vi "Pockels sequence gen-lines.vi"(8 "error in (no error)":errorcluster) -> (0 "error out":errorcluster, 1 "Lines in chunk for the trigger period target (ms)":i32, 3 "Ref Scan Cycles":i32)   [LabVIEW 2017]
uses:
  Typedefs/Pockels modulation setup cluster.ctl
  Typedefs/Frame Size.ctl
  Globals/gl_Pockels control globals.vi
panel:
  in  "Use simulation input cluster below":bool
  in  "Input values cluster":T1={"Frame Size"=512, "Fill time (us)"=24.5, "Dwell time (us)"=0.1} {"Dwell time (us)" format="%#_13g"; "Fill time (us)" format="%#_13g"; "Frame Size" items=["100X100"=100, "128X128"=128, "200X200"=200, "256X256"=256, "512X512"=512, "1024x1024"=1024, "2048x2048"=2048]}
  out "time between reference triggers (ms)":dbl[](array[numeric])
  out "Time for main img line (ms)":dbl
  out "time length of each chunk (ms)":dbl[](array[numeric])
  out "Number of lines in each chunk":i32[](array[numeric]) format="%.0f lines each"
  out "Chunks":i32[](array[numeric]) format="%.0f chunks of"
  out "Adjusted time between ref \ntriggers sent to the FPGA (ms)":dbl format="%#_10g"
  out "Actual resulting time between ref triggers (ms)":dbl format="%#_10g"
  # "INPUTS"
  # "INFORMATION"
  # "Possible combinations resulting in a number of chunks with equal number of lines"
  # "+ Time for ref image"
  # "OUTPUTS"
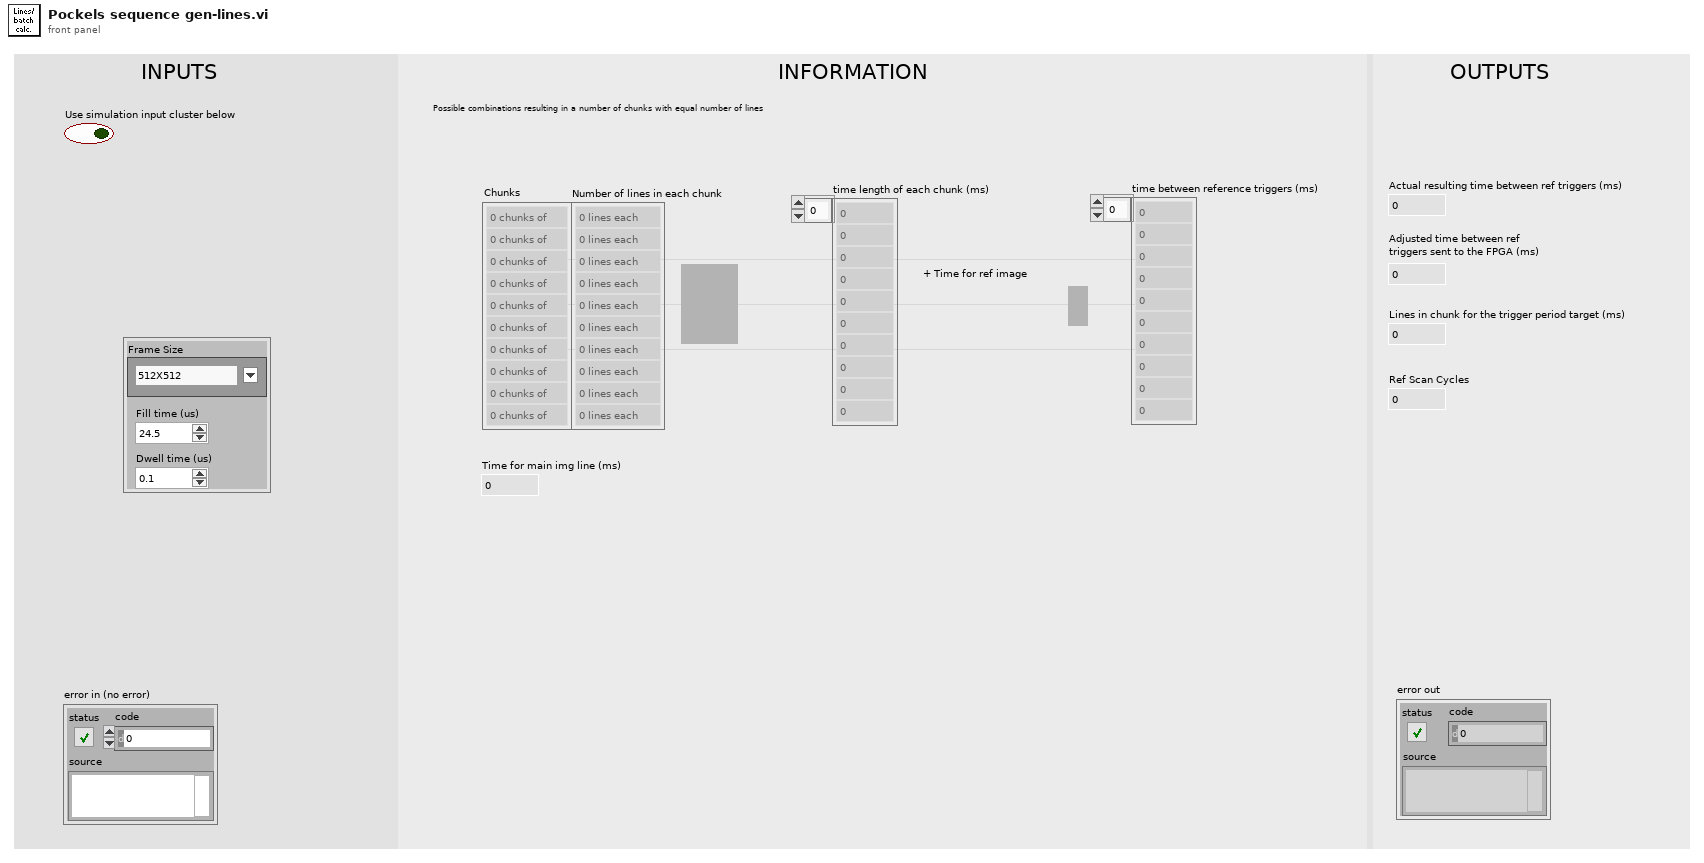
[diagram p1: front panel]
types:
  T1 = typedef "Pockels modulation setup cluster.ctl" = cluster{"Frame Size":T2, "Fill time (us)":dbl, "Dwell time (us)":dbl}
  T2 = typedef "Frame Size.ctl" = u16
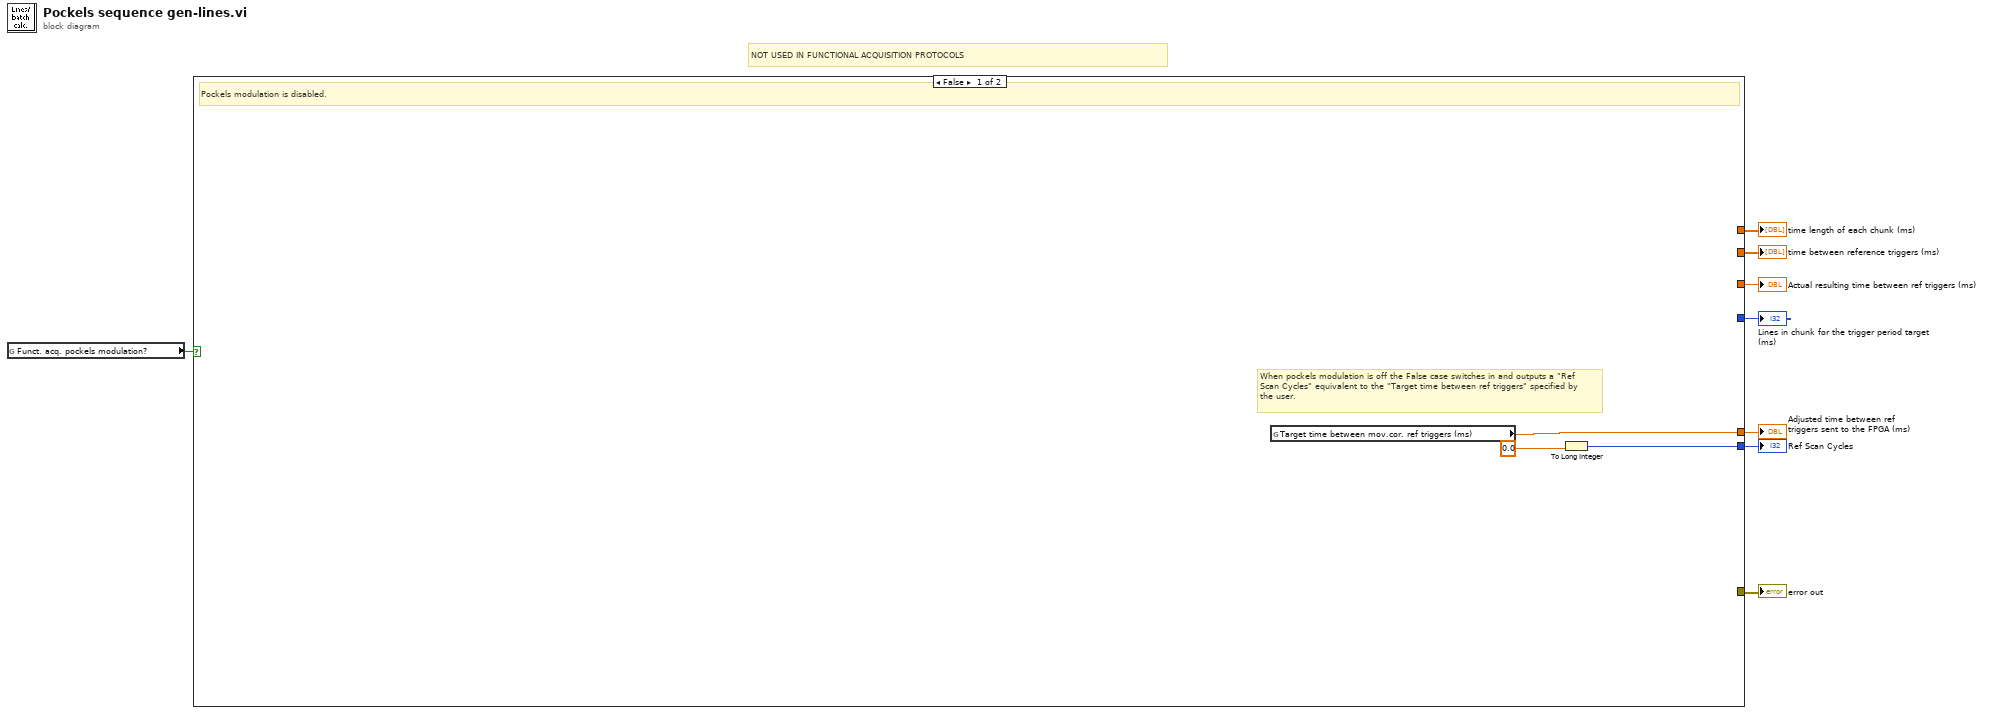
[diagram p0: block diagram]
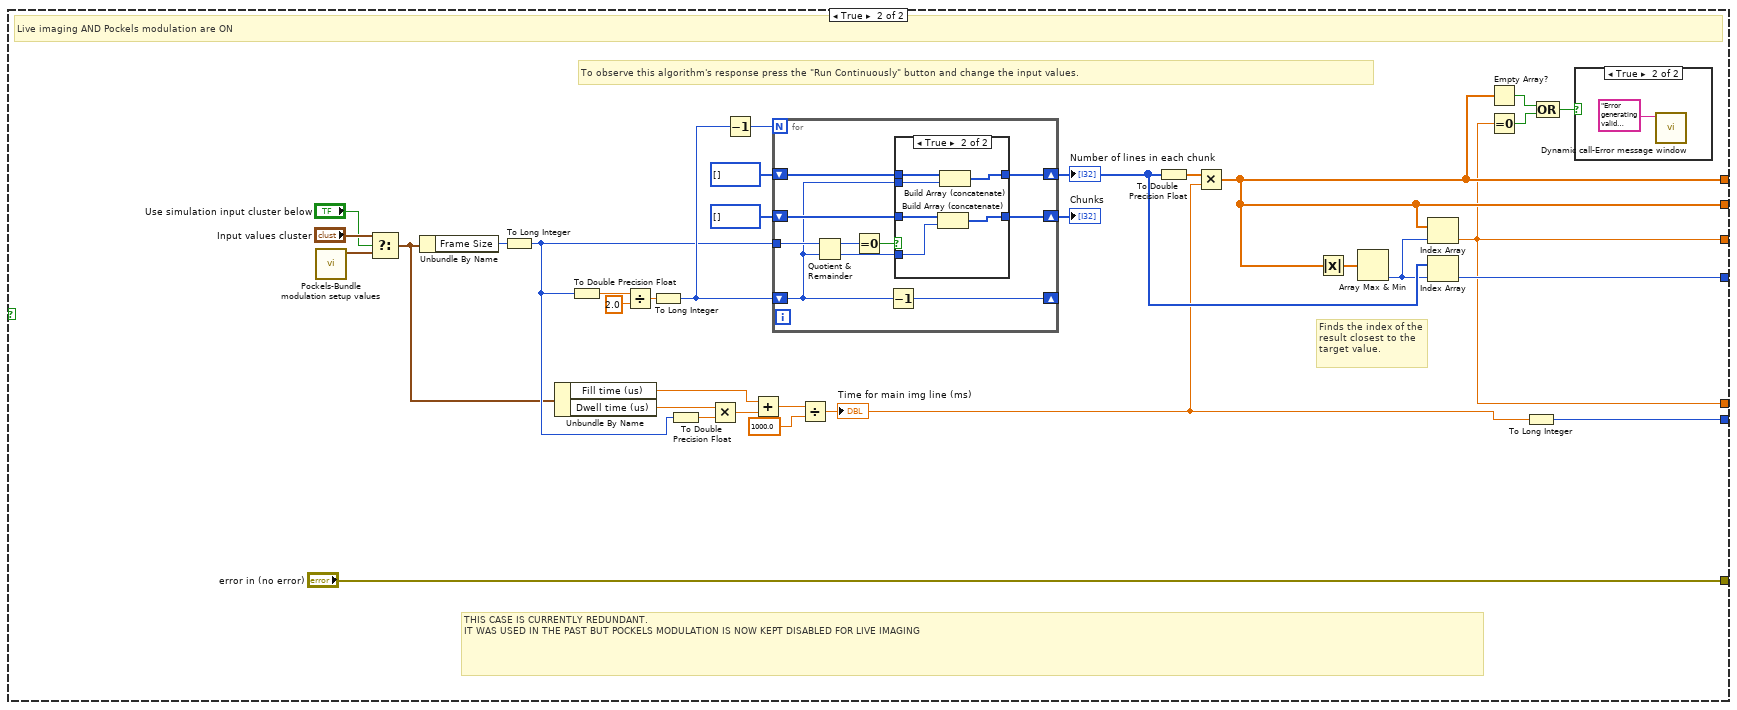
[diagram p2: hidden frame]
diagram:
  # "NOT USED IN FUNCTIONAL ACQUISITION PROTOCOLS"
  n1 = global read "gl_Pockels control globals.vi" "Funct. acq. pockels modulation?"() -> (w1:bool)
  n2 = case shown="False" w1 {
    tunnel: [_ w31] -> w8
    tunnel: [_ w14] -> w7
    tunnel: [w10 w13] -> w6
    tunnel: [w11 w23] -> w5
    tunnel: [_ w13] -> w4
    tunnel: [_ w14] -> w3
    tunnel: [_ "error in (no error)"] -> w2
    frame False {
      # "When pockels modulation is off the False case switches in and outputs a \"Ref Scan Cycles\" equivalent to the \"Target time between ref triggers\" specified by the user."
      # "Pockels modulation is disabled."
      n3 = global read "gl_Pockels control globals.vi" "Target time between mov.cor. ref triggers (ms)"() -> (w10:dbl)
      n4 = To Long Integer(number=0.0 ("Time for main img line OR for a single POI (ms)")) -> (32bit integer=w11:i32)
    }
    frame True {
      # "THIS CASE IS CURRENTLY REDUNDANT.\nIT WAS USED IN THE PAST BUT POCKELS MODULATION IS NOW KEPT DISABLED FOR LIVE IMAGING"
      # "To observe this algorithm's response press the \"Run Continuously\" button and change the input values."
      # "Finds the index of the result closest to the target value."
      # "Live imaging AND Pockels modulation are ON"
      n5 = call "Pockels-Bundle modulation setup values.vi"() -> ("Pockels modul. setup cluster"=w22:T1)  [unwired: 11 in]
      n6 = Select(t="Input values cluster", s="Use simulation input cluster below", f=w22) -> (s? t:f=w20:T1)
      n7 = Unbundle By Name(w20) -> ("Frame Size"=w26:T2)
      n8 = To Long Integer(number=w26) -> (32bit integer=w28:i32)
      n9 = Unbundle By Name(w20) -> ("Fill time (us)"=w25:dbl, "Dwell time (us)"=w24:dbl)
      n10 = To Double Precision Float(number=w28) -> (double precision float=w42:dbl)
      n11 = Divide(x=w42, y=2.0) -> (x/y=w43:dbl)
      n12 = To Long Integer(number=w43) -> (32bit integer=w41:i32)
      n13 = To Double Precision Float(number=w28) -> (double precision float=w36:dbl)
      n14 = Multiply(x=w24, y=w36) -> (x*y=w35:dbl)
      n15 = Decrement(x=w41) -> (x-1=w38:i32)
      n16 = Add(x=w25, y=w35) -> (x+y=w34:dbl)
      n17 = for {
        N: w38 -> [_]
        tunnel: w28 -> [w55]
        shift-right: [w54] -> _
        shift-left: w41 -> [w46]
        shift-right: [w51] -> w39
        shift-left: i32[] [] -> [w50]
        shift-right: [w48] -> w32
        shift-left: i32[] [] -> [w49]
        n18 = Quotient & Remainder(x=w55, y=w46) -> (x-y*floor(x/y)=w47:i32, floor(x/y)=w52:i32)
        n19 = Equal To 0?(x=w47) -> (x = 0?=w53:bool)
        n20 = Decrement(x=w46) -> (x-1=w54:i32)
        n21 = case shown="True" w53 {
          tunnel: w52 -> [_ w63]
          tunnel: [w57 w62] -> w51
          tunnel: w50 -> [w57 w61]
          tunnel: [w56 w59] -> w48
          tunnel: w49 -> [w56 w60]
          tunnel: w46 -> [_ w58]
          frame False {
          }
          frame True {
            n22 = Build Array (concatenate)(w61, w63) -> (w62:i32[])
            n23 = Build Array (concatenate)(w60, w58) -> (w59:i32[])
          }
        }
      }
      "Chunks" <- w39
      "Number of lines in each chunk" <- w32
      n24 = Divide(x=w34, y=1000.0) -> (x/y=w12:dbl)
      "Time for main img line (ms)" <- w12
      n25 = To Double Precision Float(number=w32) -> (double precision float=w27:dbl[])
      n26 = Multiply(x=w27, y=w12) -> (x*y=w14:dbl[])
      n27 = Absolute Value(x=w14) -> (abs(x)=w30:dbl[])
      n28 = Array Max & Min(array=w30) -> (min index (indices)=w29:i32)  [unwired: 3 out]
      n29 = Index Array(array=w14, index=w29) -> (element=w13:dbl)
      n30 = Index Array(array=w32, index=w29) -> (element=w31:i32)
      n31 = Empty Array?(array=w14) -> (empty?=w18:bool)
      n32 = Equal To 0?(x=w13) -> (x = 0?=w17:bool)
      n33 = To Long Integer(number=w12) -> (32bit integer=w23:i32)
      n34 = Compound Arithmetic op=OR(w18, w17) -> (w16:bool)
      n35 = case shown="True" w16 {
        frame False {
        }
        frame True {
          n36 = call "Dynamic call-Error message window.vi"("Error Message"="Error generating valid movement correction pockels modulation AO sequence.") -> ()  [unwired: 10 in, 1 out]
        }
      }
    }
  }
  "time length of each chunk (ms)" <- w3
  "time between reference triggers (ms)" <- w7
  "Lines in chunk for the trigger period target (ms)" <- w8
  "Actual resulting time between ref triggers (ms)" <- w4
  "Adjusted time between ref \ntriggers sent to the FPGA (ms)" <- w6
  "Ref Scan Cycles" <- w5
  "error out" <- w2
